vi "test Major Frame Start.vi"(8 "error in (no error)":errorcluster, 11 "BC Major Frame in":refnum<class "BC Major Frame.lvclass">) -> (0 "error out":errorcluster, 3 "BC Major Frame out":refnum<class "BC Major Frame.lvclass">)   [LabVIEW 2016, in "BC Major Frame.lvclass"]
uses:
  BC Major Frame.lvclass
  Frames & Messages/TypeDefs/BC Op Codes - Verbose.ctl
  Frames & Messages/TypeDefs/BC Condition Codes.ctl
  PPLs/FPGA Interface.lvlibp/FPGA Interface/FPGA Interface.lvclass
  BCI-1553 API.lvlib
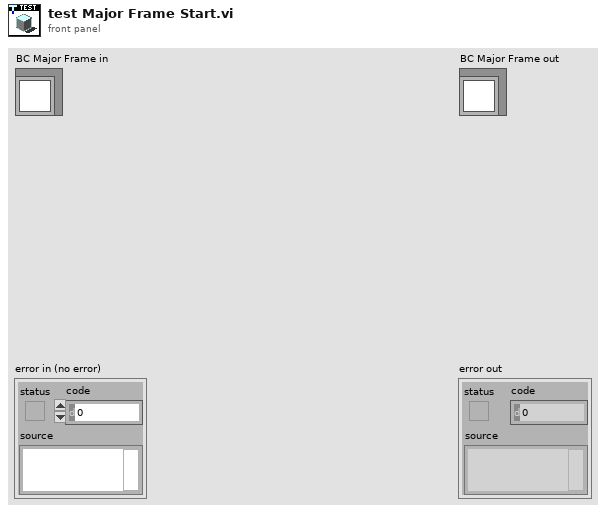
[diagram p1: front panel]
types:
  T1 = typedef "BCI-1553 API.lvlib/BC Op Codes - Verbose.ctl" = enum16{"EXECUTE MSG", "EXECUTE MSG GO", "JUMP", "CALL SUBROUTINE", "RETURN", "INTERRUPT REQUEST", "HALT", "DELAY", "WAIT FRAME TIMER = 0", "COMPARE FRAME TIMER", "COMPARE MSG TIMER", "LOAD TIME TAG CTR", "LOAD TIME TAG CTR HI", "LOAD FRAME TIMER", "START FRAME TIMER", "PUSH TIME TAG COUNT", "PUSH TIME TAG COUNT HI", "PUSH TIME TAG COUNT BOTH", "PUSH BLOCK STATUS WORD", "PUSH CURRENT VALUE", "PUSH INDIRECT", "WAIT EXT TRIGGER", "EXECUTE AND FLIP", "EXECUTE, FLIP, GO", "WRITE VALUE TO WMI", "WRITE VALUE TO MEM", "DECREMENT RAM, SKIP", "FLAG"}
  T2 = typedef "BCI-1553 API.lvlib/BC Condition Codes.ctl" = enum16{"GP0 == 1 || LT", "GP1 == 1 || NE", "GP2 == 1", "GP3 == 1", "GP4 == 1", "GP5 == 1", "GP6 == 1", "GP7 == 1", "NORESP", "FMTERR", "GOODBLOCK", "MSKSTATSET", "BADMSG", "1RETRY", "2RETRY", "ALWAYS"}
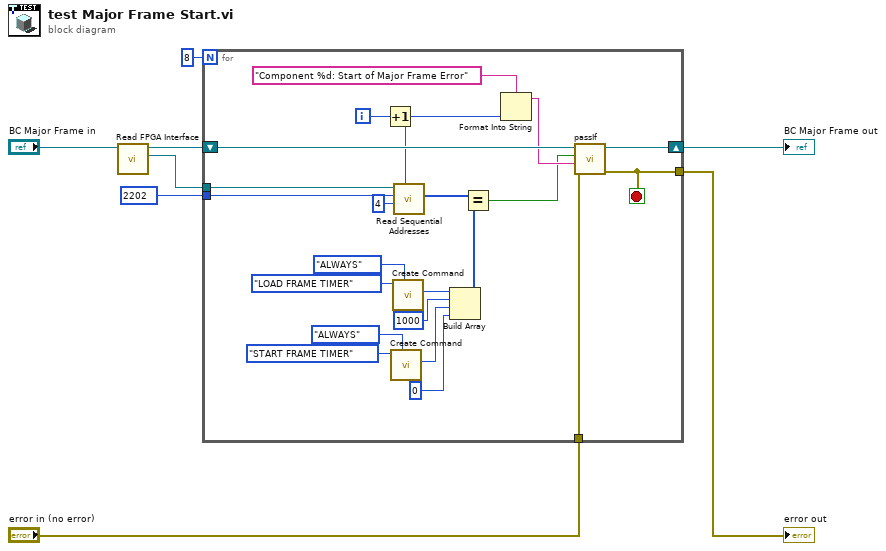
[diagram p0: block diagram]
diagram:
  n1 = call-dynamic "Read FPGA Interface.vi"("1553 Test in"="BC Major Frame in") -> ("FPGA Interface"=w5:refnum<class "FPGA Interface.lvclass">, "1553 Test out"=w7:refnum<class "BC Major Frame.lvclass">)  [unwired: 8 in, 1 out]
  n2 = for {
    N: 8 -> [_]
    shift-right: [w30] -> w6
    shift-left: w7 -> [w29]
    tunnel: w5 -> [w28]
    tunnel: u16 2202 -> [w24]
    tunnel: "error in (no error)" -> [w10]
    tunnel: [w9] -> w2
    i -> [w26]
    stop <- w9 stop-if-true
    n3 = Increment(x=w26) -> (x+1=w22:i32)
    n4 = call "Create Command.vi"("Condition"=BC_Condition_Codes."ALWAYS", "Op Code"=BC_Op_Codes_-_Verbose."START FRAME TIMER") -> ("Instruction"=w15:u16)  [unwired: 8 in, 1 out]
    n5 = call "Create Command.vi"("Condition"=BC_Condition_Codes."ALWAYS", "Op Code"=BC_Op_Codes_-_Verbose."LOAD FRAME TIMER") -> ("Instruction"=w17:u16)  [unwired: 8 in, 1 out]
    n6 = call-dynamic "Read Sequential Addresses.vi"("Target IC (1-8)"=w22, "Addresses to Read"=u16 4, "Starting Address"=w24, "FPGA Interface in"=w28) -> ("Data"=w12:u16[])  [unwired: 6 in, 1 out]
    n7 = Build Array(w17, u16 1000 ("x"), w15, u16 0 ("x")) -> (w13:u16[])
    n8 = Equal?(x=w12, y=w13) -> (x = y?=w11:bool)
    n9 = Format Into String(format string="Component %d: Start of Major Frame Error" ("custom report message (\"\")"), w22) -> (resulting string=w25:string)  [unwired: 2 in, 1 out]
    n10 = call-dynamic "passIf.vi"("error in (no error)"=w10, "message (\"\")"=w25, "pass"=w11, "TestCase in"=w29) -> ("error out"=w9:errorcluster, "TestCase out"=w30:refnum<class "BC Major Frame.lvclass">)  [unwired: 6 in]
  }
  "error out" <- w2
  "BC Major Frame out" <- w6
